vi "mm2units.vi"(8 "lambda (nm)":dbl, 10 "target units":string(combo), 11 "raw position (mm)":dbl) -> (3 "position in units":dbl)   [LabVIEW 2023]
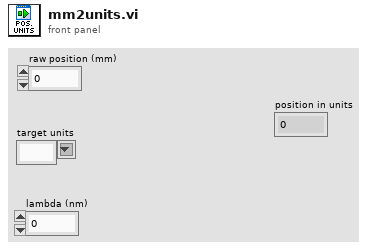
[diagram p1: front panel]
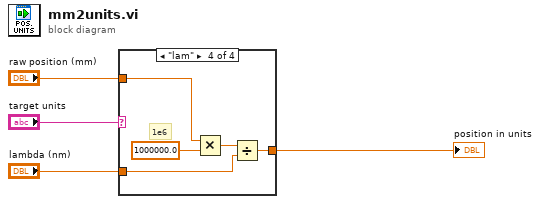
[diagram p0: block diagram]
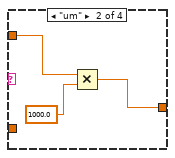
[diagram p3: hidden frame]
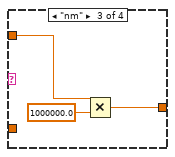
[diagram p4: hidden frame]
diagram:
  n1 = case shown="\"lam\"" "target units" {
    tunnel: [w5 w6 w9 w13] -> w1
    tunnel: "raw position (mm)" -> [w5 w7 w10 w14]
    tunnel: "lambda (nm)" -> [_ _ _ w12]
    frame "mm", Default {
    }
    frame "um" {
      n2 = Multiply(x=w7, y=1000.0) -> (x*y=w6:dbl)
    }
    frame "nm" {
      n3 = Multiply(x=w10, y=1000000.0) -> (x*y=w9:dbl)
    }
    frame "lam" {
      # "1e6"
      n4 = Multiply(x=w14, y=1000000.0) -> (x*y=w16:dbl)
      n5 = Divide(x=w16, y=w12) -> (x/y=w13:dbl)
    }
  }
  "position in units" <- w1
